vi "SVM Cross-Validate ONE_CLASS.vi"(6 "Nr fold":i32 caption="Nr fold (LOO)", 7 "Options":T6={"cache_size"=200.0, "eps"=0.001, "shrinking"=TRUE, "probability"=FALSE}, 8 "error in (no error)":errorcluster, 9 "nu":T1=0.5 caption="nu (0,5)", 10 "Kernel":T4, 11 "Problem":T2) -> (0 "error out":errorcluster, 3 "Target":dbl[](array[numeric]) caption="Target (Predicted labels)")   [LabVIEW 2015]
doc: "This function conducts cross validation. Data are separated to nr_fold folds. Under given parameters sequentially each fold is validated using the model from training the remaining. Predicted labels (of all prob's instances) in the validation process are stored in the array called target.\n\nThe default number of folds uses Leave-One-Out cross-validation (LOO)."
uses:
  Controls/Options Training.ctl
  Controls/Kernel.ctl
  Wrapper API/Controls/svm_kernel_type.ctl
  Wrapper API/Controls/svm_problem.ctl
  Wrapper API/Controls/svm_node.ctl
  Controls/Parameters ONE_CLASS.ctl
  Wrapper API/Controls/svm_parameter.ctl
  Wrapper API/Controls/svm_type.ctl
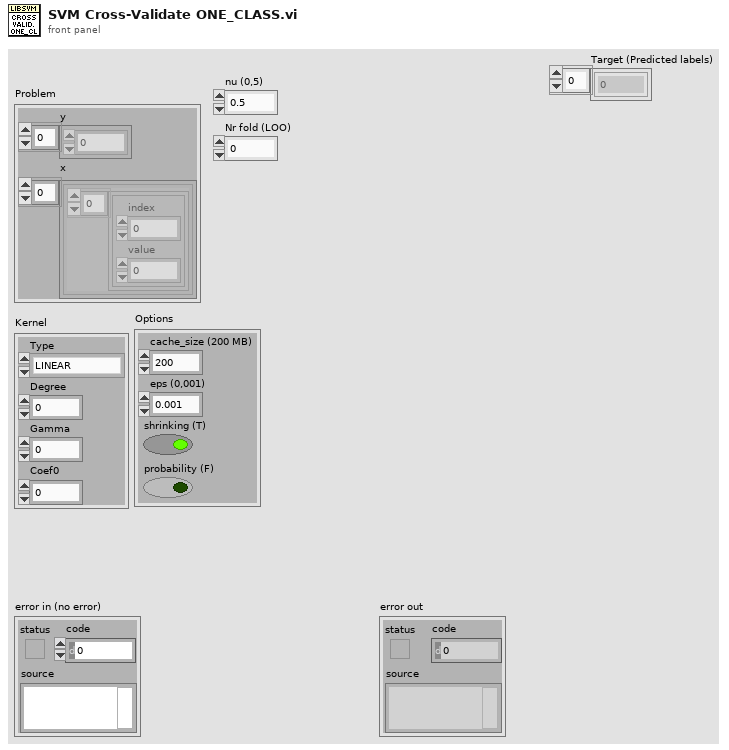
[diagram p1: front panel]
types:
  T1 = typedef "Parameters ONE_CLASS.ctl" = dbl
  T2 = typedef "svm_problem.ctl" = cluster{"y":dbl[], "x":cluster{T3[]}[]}
  T3 = typedef "svm_node.ctl" = cluster{"index":i32, "value":dbl}
  T4 = typedef "Kernel.ctl" = cluster{"Type":T5, "Degree":i32, "Gamma":dbl, "Coef0":dbl}
  T5 = typedef "svm_kernel_type.ctl" = enum32{"LINEAR", "POLY", "RBF", "SIGMOID", "PRECOMPUTED"}
  T6 = typedef "Options Training.ctl" = cluster{"cache_size":dbl, "eps":dbl, "shrinking":bool, "probability":bool}
  T7 = typedef "svm_type.ctl" = enum32{"C_SVC", "NU_SVC", "ONE_CLASS", "EPSILON_SVR", "NU_SVR"}
  T8 = typedef "svm_parameter.ctl" = cluster{"svm_type":T7, "kernel_type":T5, "degree":i32, "gamma":dbl, "coef0":dbl, "cache_size":dbl, "eps":dbl, "C":dbl, "weight_label":i32[], "weight":dbl[], "nu":dbl, "p":dbl, "shrinking":bool, "probability":bool}
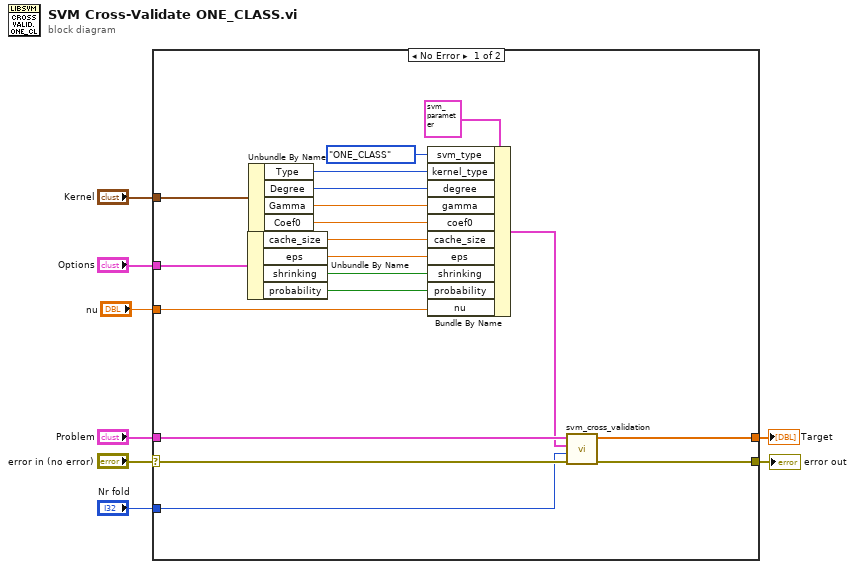
[diagram p0: block diagram]
diagram:
  n1 = case shown="No Error" "error in (no error)" {
    selector: "error in (no error)" -> [w11 w28]
    tunnel: [w12 w28] -> w8
    tunnel: "Problem" -> [w14 _]
    tunnel: "Kernel" -> [w26 _]
    tunnel: [w13 _] -> w2
    tunnel: "Options" -> [w18 _]
    tunnel: "nu" -> [w15 _]
    tunnel: "Nr fold" -> [w9 _]
    frame No Error {
      n2 = Unbundle By Name(w18) -> ("cache_size"=w20:dbl, "eps"=w19:dbl, "shrinking"=w17:bool, "probability"=w16:bool)
      n3 = Unbundle By Name(w26) -> ("Type"=w25:T5, "Degree"=w24:i32, "Gamma"=w23:dbl, "Coef0"=w22:dbl)
      n4 = Bundle By Name(cluster=T8 {"svm_type"=enum."C_SVC", "kernel_type"=enum."LINEAR", "degree"=0, "gamma"=0.0, "coef0"=0.0, "cache_size"=0.0, "eps"=0.0, "C"=0.0, "weight_label"=[], "weight"=[], "nu"=0.0, "p"=0.0, "shrinking"=FALSE, "probability"=FALSE} ("svm_parameter"), "svm_type"=svm_type."ONE_CLASS", "kernel_type"=w25, "degree"=w24, "gamma"=w23, "coef0"=w22, "cache_size"=w20, "eps"=w19, "shrinking"=w17, "probability"=w16, "nu"=w15) -> (w10:T8)
      n5 = call "svm_cross_validation.vi"("error in (no error)"=w11, "Nr fold"=w9, "Parameters"=w10, "Problem"=w14) -> ("error out"=w12:errorcluster, "Target"=w13:dbl[])  [unwired: 6 in]
    }
    frame Error {
    }
  }
  "error out" <- w8
  "Target" <- w2
